vi "TCP Listener.vi"() -> ()   [LabVIEW 2019, in "Common System Tests.lvclass"]
uses:
  Common System Tests.lvclass
panel:
  out "No of messages":i32
  out "Recieved Messages":string[](array[string])
  out "current data out":string
  in  "error in (no error)":errorcluster
  out "error out":errorcluster
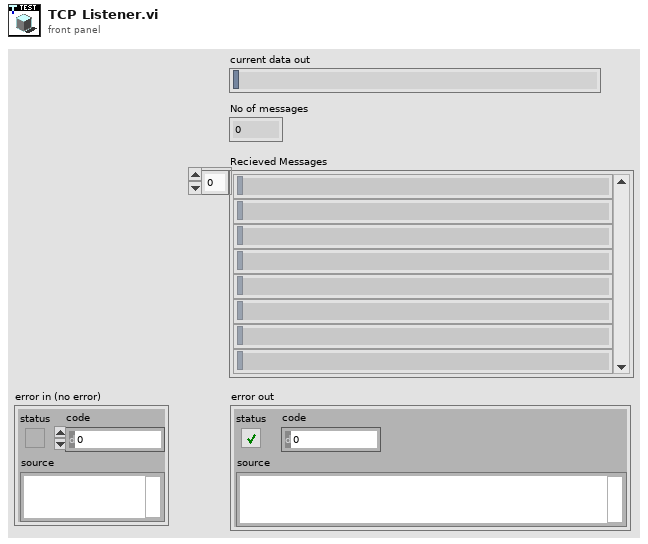
[diagram p1: front panel]
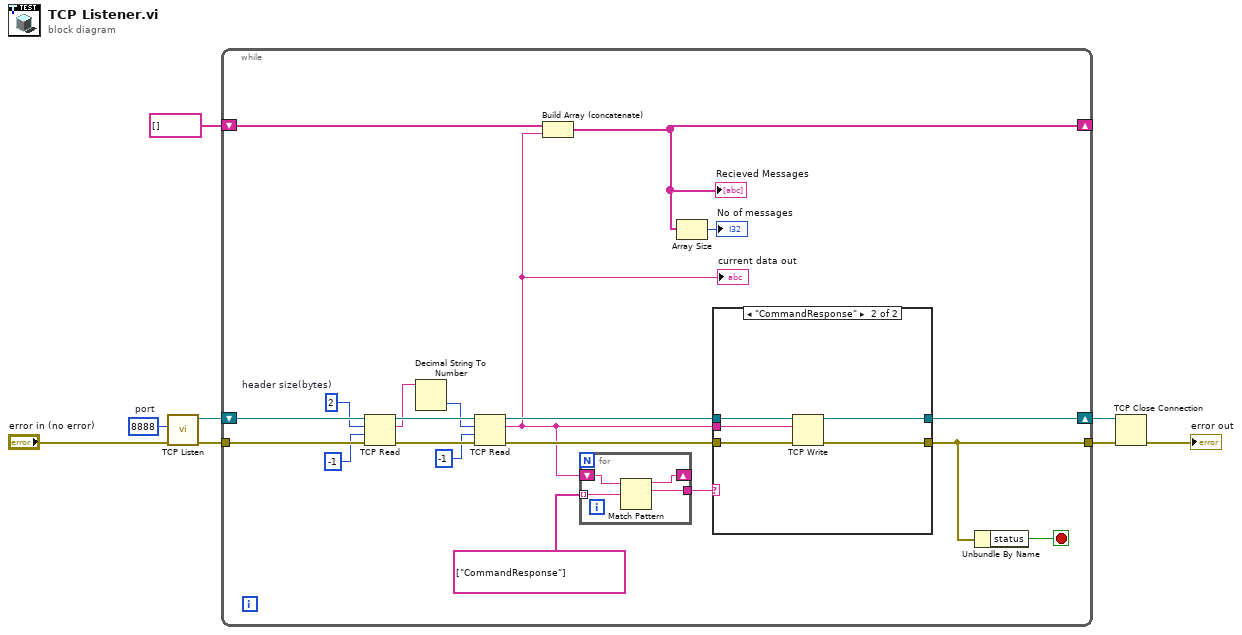
[diagram p0: block diagram]
diagram:
  w5 = u16 8888  # port
  n1 = call <vilib>:"TCP Listen.vi"("error in (no error)"="error in (no error)", "port"=w5) -> ("error out"=w3:errorcluster, "connection ID"=w4:refnum<k5>)  [unwired: 5 in, 3 out]
  n2 = while {
    shift-right: [w12] -> _
    shift-left: string[] [] -> [w26]
    shift-right: [w14] -> w8
    shift-left: w4 -> [w28]
    tunnel: w3 -> [w27]
    tunnel: [w16] -> w7
    stop <- w17 stop-if-true
    w25 = 2  # header size(bytes)
    n3 = TCP Read(connection ID=w28, bytes to read=w25, error in (no error)=w27, 9:-1 ("timeout ms (25000)")) -> (connection ID out=w22:refnum<k5>, data out=w21:string, error out=w23:errorcluster)  [unwired: 1 in]
    n4 = Decimal String To Number(string=w21) -> (number=w20:i32)  [unwired: 2 in, 1 out]
    n5 = TCP Read(connection ID=w22, bytes to read=w20, error in (no error)=w23, 9:-1 ("timeout ms (25000)")) -> (connection ID out=w15:refnum<k5>, data out=w9:string, error out=w18:errorcluster)  [unwired: 1 in]
    "current data out" <- w9
    n6 = Build Array (concatenate)(w26, w9) -> (w12:string[])
    "Recieved Messages" <- w12
    n7 = for {
      tunnel: string[] ["CommandResponse"] ("regular expression") -> [w31] mode=indexing
      tunnel: [w32] -> w11
      shift-right: [w29] -> _
      shift-left: w9 -> [w30]
      n8 = Match Pattern(string=w30, regular expression=w31) -> (before substring=w29:string, match substring=w32:string)  [unwired: 1 in, 2 out]
    }
    n9 = Array Size(array=w12) -> (size(s)=→"No of messages":i32)
    n10 = case shown="\"CommandResponse\"" w11 {
      tunnel: w18 -> [w34 w39]
      tunnel: [w34 w38] -> w16
      tunnel: w15 -> [w33 w37]
      tunnel: [w33 w36] -> w14
      tunnel: w9 -> [_ w35]
      frame "CommandOnly", Default {
      }
      frame "CommandResponse" {
        n11 = TCP Write(connection ID=w37, data in=w35, error in (no error)=w39) -> (connection ID out=w36:refnum<k5>, error out=w38:errorcluster)  [unwired: 1 in, 1 out]
      }
    }
    n12 = Unbundle By Name(w16) -> ("status"=w17:bool)
  }
  n13 = TCP Close Connection(connection ID=w8, error in (no error)=w7) -> (error out=→"error out":errorcluster)  [unwired: 1 in, 1 out]
